vi "merFISH_count_probes.vi"(4 "MCListbox Refnum":refnum<vi>, 5 "error in":errorcluster) -> (0 "error out":errorcluster, 3 "At least one probe?":bool)   [LabVIEW 2015]
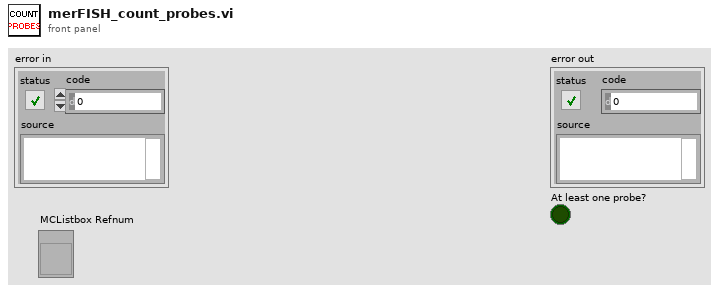
[diagram p1: front panel]
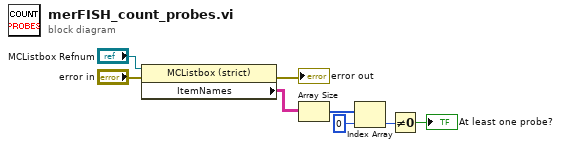
[diagram p0: block diagram]
diagram:
  n1 = property class="MCListbox (strict)"(reference="MCListbox Refnum", error in="error in") -> (error out=→"error out":errorcluster, "ItemNames"=w8:string[][])  [unwired: 1 out]
  n2 = Array Size(array=w8) -> (size(s)=w4:i32[])
  n3 = Index Array(array=w4, index=0) -> (element=w2:i32)
  n4 = Not Equal To 0?(x=w2) -> (x != 0?=→"At least one probe?":bool)
